vi "Decode Error.vi"(8 "error in (no error)":errorcluster, 11 "VISA resource name":refnum<visa-resource-name>) -> (0 "error out":errorcluster, 2 "Error Message":string, 3 "VISA resource name out":refnum<visa-resource-name>)   [LabVIEW 2019, in "Lake Shore 372.lvlib"]
doc: "Called by the 350 Error Query VI. It's function is to query the 350 Status Byte and decode errors if the Status Byte reports errors are present. \n\nNote that the calling VI checks the Status Byte in the case of a timeout error. If the calling VI indicates the Status Byte is already reporting errors, this VI will not query the Status Byte again, it will go straight to the process of decoding errors.\n\nThe following conditions will be returned as errors in the Error Out cluster:\n<B>Processor Communication Error</B>\n<B>Query Error</B>\n<B>Execution Error</B>\n<B>Command Error</B>\n<B>Calibration Error</B>\n\nThe following conditions will be returned as warnings in the Error Out cluster:\n<B>Sensor Alarming</B>\n<B>Invalid Reading</B>\n<B>Temperature Underrange</B>\n<B>Temperature Overrange</B>\n<B>Sensor Units Zero</B>\n<B>Sensor Units Overrange</B>"
uses:
  Lake Shore 372.lvlib
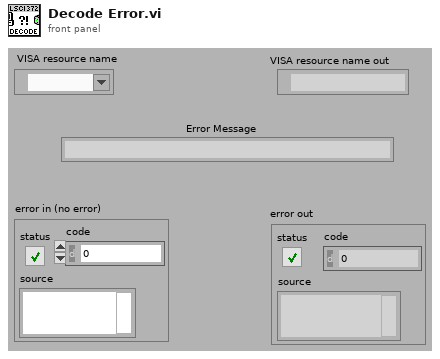
[diagram p1: front panel]
types:
  T1 = enum16{"Query STB", "Check bit 3", "Check bit 4", "Check bit 5", "Check ESR", "ESR Error Handling", "Input Error Handling", "Output Error"}
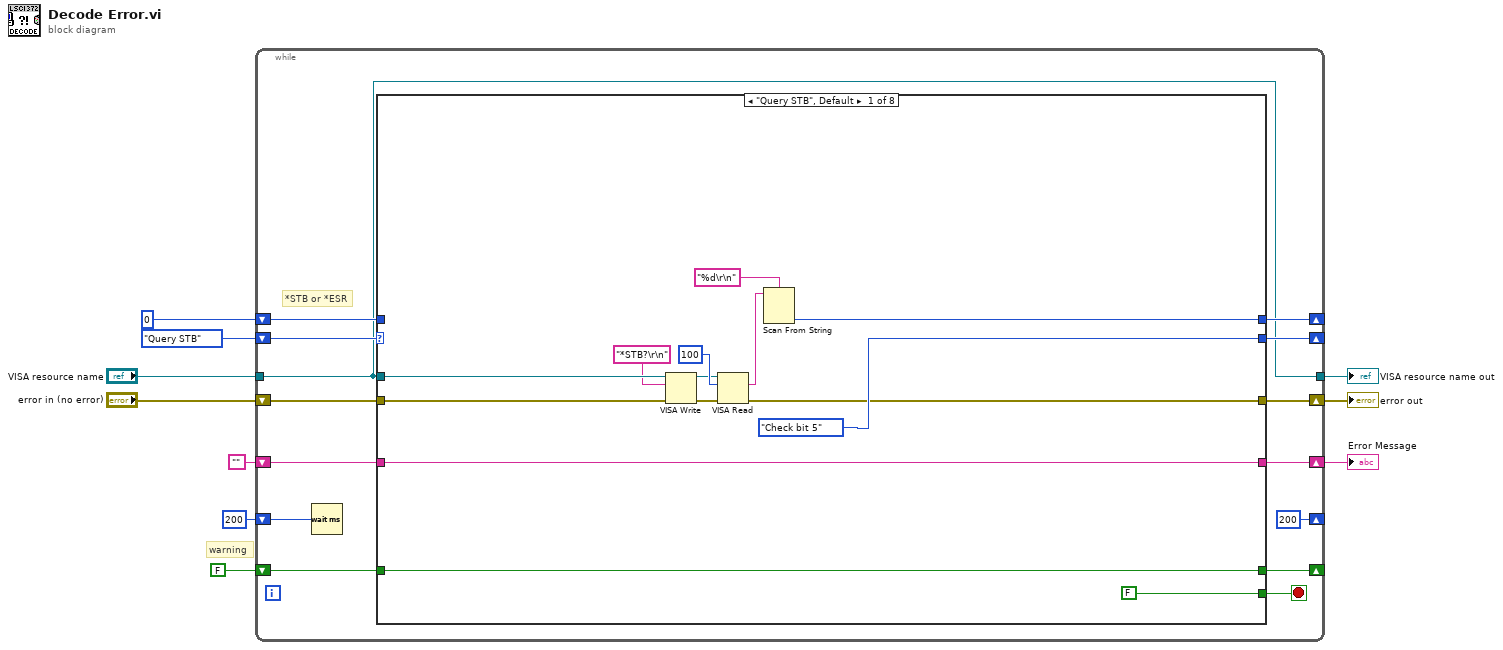
[diagram p0: block diagram]
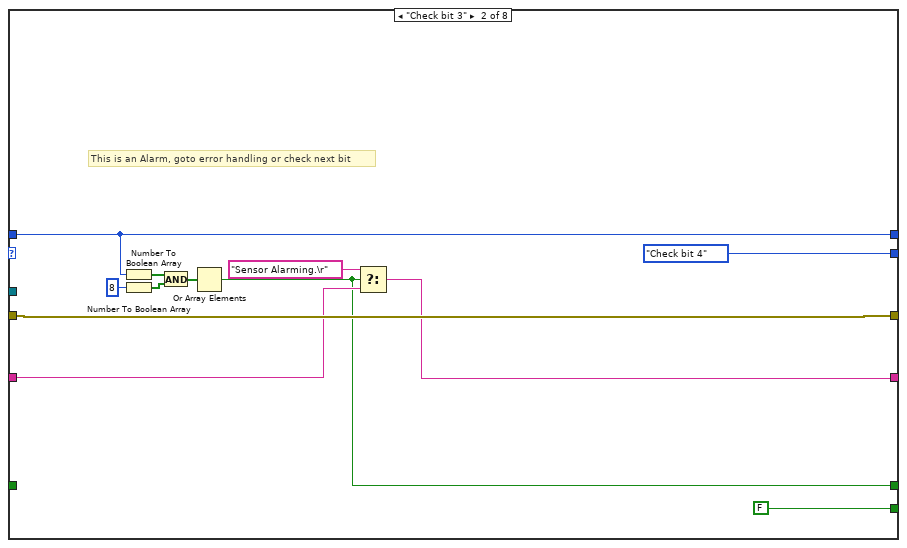
[diagram p2: hidden frame]
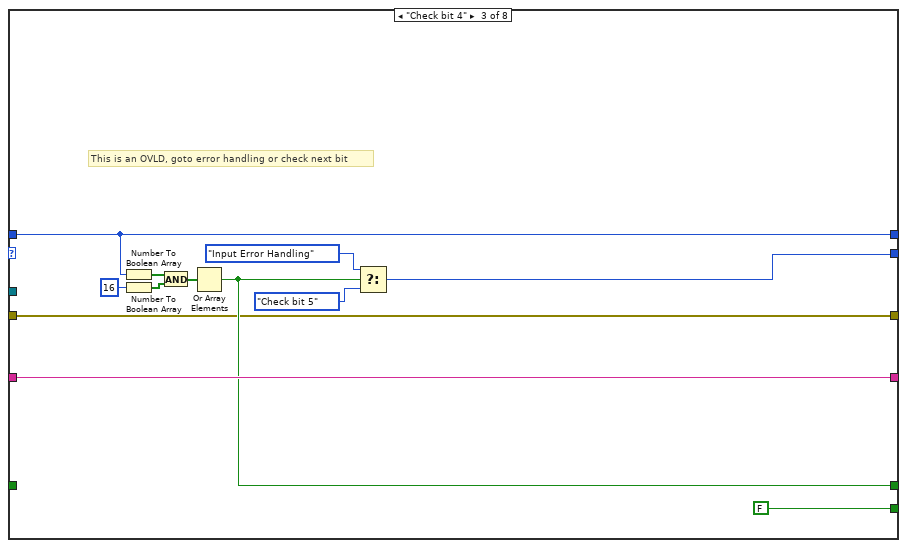
[diagram p3: hidden frame]
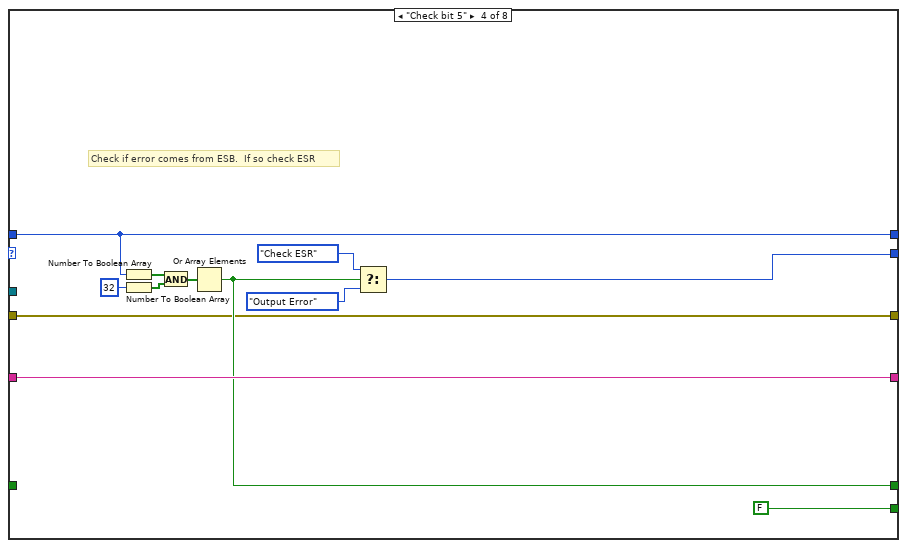
[diagram p4: hidden frame]
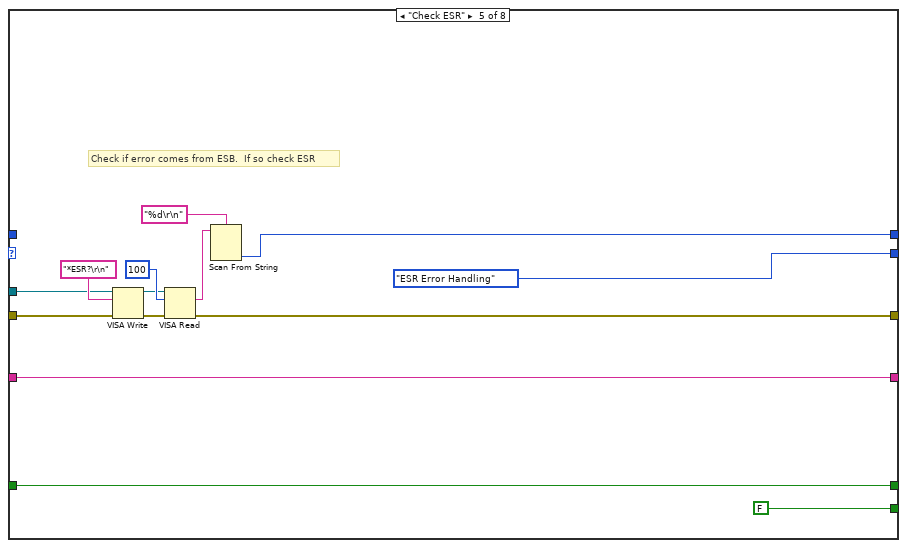
[diagram p5: hidden frame]
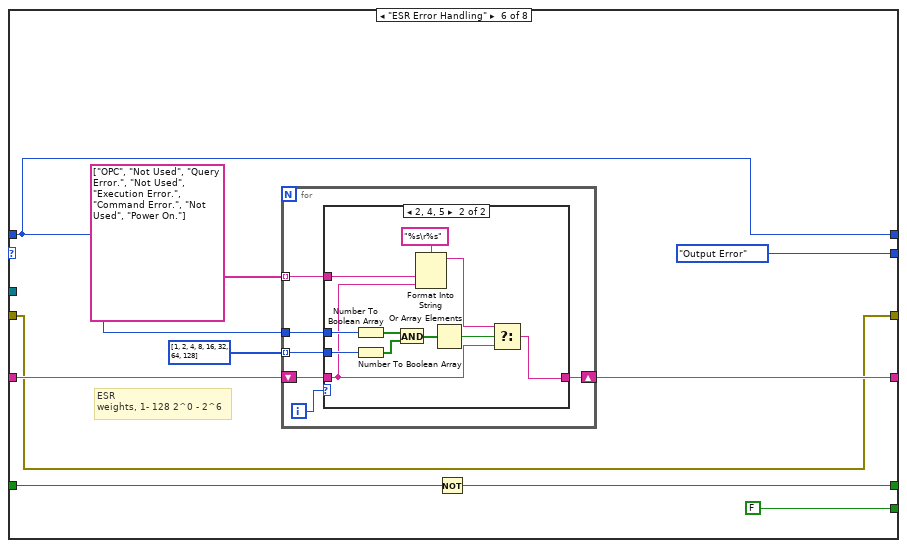
[diagram p6: hidden frame]
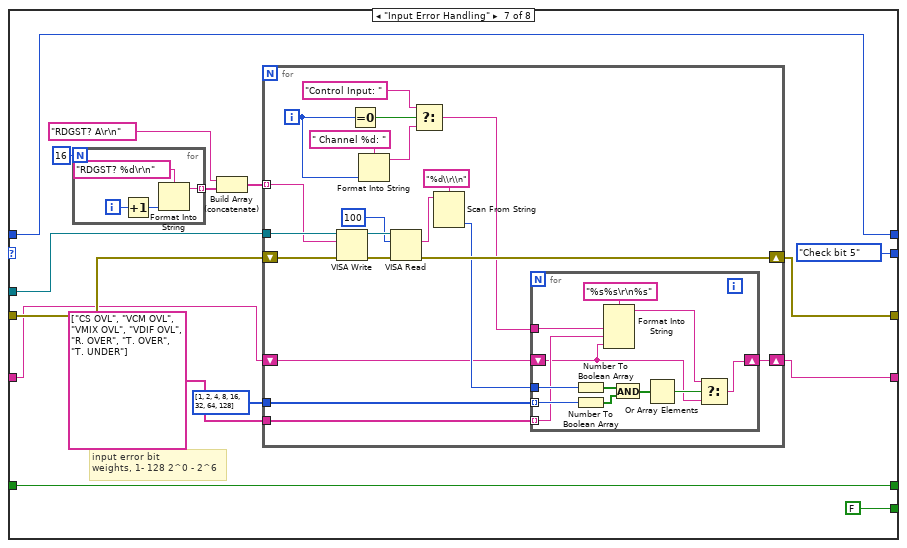
[diagram p8: hidden frame]
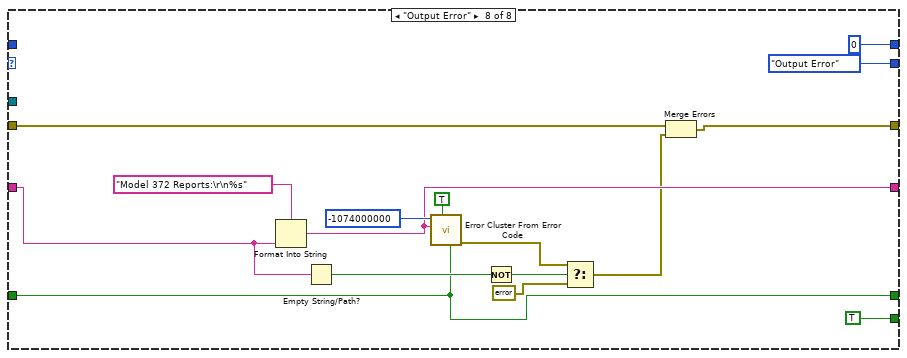
[diagram p9: hidden frame]
diagram:
  # "warning"
  n1 = while {
    shift-right: [w23] -> _
    shift-left: 0 -> [w22]
    shift-right: [w21] -> _
    shift-left: T1."Query STB" -> [w24]
    shift-right: [w19] -> w6
    shift-left: "" -> [w18]
    shift-right: [w16] -> _
    shift-left: FALSE -> [w17]
    tunnel: "VISA resource name" -> [w13]
    shift-right: [w14] -> w3
    shift-left: "error in (no error)" -> [w15]
    tunnel: [w13] -> w2
    shift-right: [u32 200 ("milliseconds to wait")] -> _
    shift-left: u32 200 ("milliseconds to wait") -> [w12]
    stop <- w20 stop-if-true
    # "*STB or *ESR"
    n2 = Wait (ms)(milliseconds to wait=w12) -> ()  [unwired: 1 out]
    n3 = case shown="\"Query STB\", Default" w24 {
      tunnel: [w38 w46 w58 w70 w82 w96 w131 0] -> w23
      tunnel: w22 -> [_ w46 w58 w70 _ w96 w131 _]
      tunnel: [T1."Check bit 5" T1."Check bit 4" w55 w67 T1."ESR Error Handling" T1."Output Error" T1."Check bit 5" T1."Output Error"] -> w21
      tunnel: [FALSE FALSE FALSE FALSE FALSE FALSE FALSE TRUE] -> w20
      tunnel: [w36 w41 w53 w65 w80 w93 w121 w172] -> w19
      tunnel: w18 -> [w36 w42 w53 w65 w80 w92 w117 w173]
      tunnel: w17 -> [w34 _ _ _ w78 w91 w128 w171]
      tunnel: [w34 w39 w52 w64 w78 w90 w128 w171] -> w16
      tunnel: w13 -> [w33 _ _ _ w77 _ w120 _]
      tunnel: w15 -> [w32 w44 w51 w63 w76 w89 w119 w169]
      tunnel: [w31 w44 w51 w63 w75 w89 w118 w168] -> w14
      frame "Query STB", Default {
        n4 = VISA Write(VISA resource name=w33, write buffer="*STB?\r\n", error in (no error)=w32) -> (VISA resource name out=w27:refnum<visa-resource-name>, error out=w26:errorcluster)  [unwired: 1 out]
        n5 = VISA Read(VISA resource name=w27, byte count=u32 100, error in (no error)=w26) -> (read buffer=w30:string, error out=w31:errorcluster)  [unwired: 2 out]
        n6 = Scan From String(format string="%d\r\n", input string=w30) -> (output 1=w38:i32)  [unwired: 3 in, 3 out]
      }
      frame "Check bit 3" {
        # "This is an Alarm, goto error handling or check next bit"
        n7 = Number To Boolean Array(number=w46) -> (Boolean array=w47:bool[])
        n8 = Number To Boolean Array(number=8 ("index")) -> (Boolean array=w48:bool[])
        n9 = And(x=w47, y=w48) -> (x .and. y?=w50:bool[])
        n10 = Or Array Elements(Boolean array=w50) -> (logical OR=w39:bool)
        n11 = Select(t="Sensor Alarming.\r", s=w39, f=w42) -> (s? t:f=w41:string)
      }
      frame "Check bit 4" {
        # "This is an OVLD, goto error handling or check next bit"
        n12 = Number To Boolean Array(number=w58) -> (Boolean array=w59:bool[])
        n13 = Number To Boolean Array(number=16 ("index")) -> (Boolean array=w60:bool[])
        n14 = And(x=w59, y=w60) -> (x .and. y?=w62:bool[])
        n15 = Or Array Elements(Boolean array=w62) -> (logical OR=w52:bool)
        n16 = Select(t=T1."Input Error Handling", s=w52, f=T1."Check bit 5") -> (s? t:f=w55:T1)
      }
      frame "Check bit 5" {
        # "Check if error comes from ESB.  If so check ESR"
        n17 = Number To Boolean Array(number=w70) -> (Boolean array=w71:bool[])
        n18 = Number To Boolean Array(number=32 ("index")) -> (Boolean array=w72:bool[])
        n19 = And(x=w71, y=w72) -> (x .and. y?=w74:bool[])
        n20 = Or Array Elements(Boolean array=w74) -> (logical OR=w64:bool)
        n21 = Select(t=T1."Check ESR", s=w64, f=T1."Output Error") -> (s? t:f=w67:T1)
      }
      frame "Check ESR" {
        # "Check if error comes from ESB.  If so check ESR"
        n22 = VISA Write(VISA resource name=w77, write buffer="*ESR?\r\n", error in (no error)=w76) -> (VISA resource name out=w85:refnum<visa-resource-name>, error out=w84:errorcluster)  [unwired: 1 out]
        n23 = VISA Read(VISA resource name=w85, byte count=u32 100, error in (no error)=w84) -> (read buffer=w88:string, error out=w75:errorcluster)  [unwired: 2 out]
        n24 = Scan From String(format string="%d\r\n", input string=w88) -> (output 1=w82:i32)  [unwired: 3 in, 3 out]
      }
      frame "ESR Error Handling" {
        # "ESR\nweights, 1- 128 2^0 - 2^6"
        n25 = for {
          tunnel: w96 -> [w103]
          tunnel: i32[] [1, 2, 4, 8, 16, 32, 64, 128] -> [w102] mode=indexing
          shift-right: [w99] -> w93
          shift-left: w92 -> [w101]
          tunnel: string[] ["OPC", "Not Used", "Query Error.", "Not Used", "Execution Error.", "Command Error.", "Not Used", "Power On."] -> [w100] mode=indexing
          i -> [w104]
          n26 = case shown="2, 4, 5" w104 {
            tunnel: w103 -> [_ w116]
            tunnel: w102 -> [_ w115]
            tunnel: w101 -> [w105 w108]
            tunnel: w100 -> [_ w110]
            tunnel: [w105 w107] -> w99
            frame 1, Default {
            }
            frame 2, 4, 5 {
              n27 = Number To Boolean Array(number=w116) -> (Boolean array=w114:bool[])
              n28 = Number To Boolean Array(number=w115) -> (Boolean array=w113:bool[])
              n29 = And(x=w114, y=w113) -> (x .and. y?=w112:bool[])
              n30 = Format Into String(format string="%s\r%s", w110, w108) -> (resulting string=w109:string)  [unwired: 2 in, 1 out]
              n31 = Or Array Elements(Boolean array=w112) -> (logical OR=w106:bool)
              n32 = Select(t=w109, s=w106, f=w108) -> (s? t:f=w107:string)
            }
          }
        }
        n33 = Not(x=w91) -> (.not. x?=w90:bool)
      }
      frame "Input Error Handling" {
        # "input error bit\nweights, 1- 128 2^0 - 2^6"
        n34 = for {
          N: 16 -> [_]
          tunnel: [w164] -> w126 mode=indexing
          i -> [w167]
          n35 = Increment(x=w167) -> (x+1=w166:i32)
          n36 = Format Into String(format string="RDGST? %d\r\n", w166) -> (resulting string=w164:string)  [unwired: 2 in, 1 out]
        }
        n37 = Build Array (concatenate)("RDGST? A\r\n" ("format string"), w126) -> (w124:string[])
        n38 = for {
          shift-right: [w144] -> w118
          shift-left: w119 -> [w151]
          tunnel: w124 -> [w149] mode=indexing
          tunnel: i32[] [1, 2, 4, 8, 16, 32, 64, 128] -> [w142]
          tunnel: string[] ["CS OVL", "VCM OVL", "VMIX OVL", "VDIF OVL", "R. OVER", "T. OVER", "T. UNDER"] -> [w141]
          shift-right: [w135] -> w121
          shift-left: w117 -> [w140]
          tunnel: w120 -> [w150]
          i -> [w137]
          n39 = VISA Write(VISA resource name=w150, write buffer=w149, error in (no error)=w151) -> (VISA resource name out=w147:refnum<visa-resource-name>, error out=w148:errorcluster)  [unwired: 1 out]
          n40 = Equal To 0?(x=w137) -> (x = 0?=w138:bool)
          n41 = Format Into String(format string=" Channel %d: ", w137) -> (resulting string=w136:string)  [unwired: 2 in, 1 out]
          n42 = VISA Read(VISA resource name=w147, byte count=u32 100, error in (no error)=w148) -> (read buffer=w146:string, error out=w144:errorcluster)  [unwired: 2 out]
          n43 = Select(t="Control Input: " ("format string"), s=w138, f=w136) -> (s? t:f=w132:string)
          n44 = Scan From String(format string="%d\\r\\n", input string=w146) -> (output 1=w143:i32)  [unwired: 3 in, 3 out]
          n45 = for {
            tunnel: w143 -> [w163]
            tunnel: w142 -> [w162] mode=indexing
            tunnel: w141 -> [w154] mode=indexing
            shift-right: [w157] -> w135
            shift-left: w140 -> [w153]
            tunnel: w132 -> [w155]
            n46 = Number To Boolean Array(number=w163) -> (Boolean array=w160:bool[])
            n47 = Number To Boolean Array(number=w162) -> (Boolean array=w161:bool[])
            n48 = Format Into String(format string="%s%s\r\n%s", w155, w154, w153) -> (resulting string=w152:string)  [unwired: 2 in, 1 out]
            n49 = And(x=w160, y=w161) -> (x .and. y?=w159:bool[])
            n50 = Or Array Elements(Boolean array=w159) -> (logical OR=w158:bool)
            n51 = Select(t=w152, s=w158, f=w153) -> (s? t:f=w157:string)
          }
        }
      }
      frame "Output Error" {
        n52 = Format Into String(format string="Model 372 Reports:\r\n%s", w173) -> (resulting string=w172:string)  [unwired: 2 in, 1 out]
        n53 = Empty String/Path?(string/path=w173) -> (empty?=w177:bool)
        n54 = call <vilib>:"Error Cluster From Error Code.vi"("is warning? (False)"=w171, "show call chain? (False)"=TRUE, "error message (\"\")"=w172, "error code (0)"=-1074000000 ("Code")) -> ("error out"=w180:errorcluster)  [unwired: 5 in]
        n55 = Not(x=w177) -> (.not. x?=w178:bool)
        n56 = Select(t=w180, s=w178, f=errorcluster {"status"=FALSE, "code"=0, "source"=""} ("error out")) -> (s? t:f=w170:errorcluster)
        n57 = Merge Errors(w169, w170) -> (w168:errorcluster)
      }
    }
  }
  "error out" <- w3
  "VISA resource name out" <- w2
  "Error Message" <- w6
